vi "workbook add signed vba project.vi"(8 "error in (no error)":errorcluster, 9 "signature":string, 10 "vba_project":string, 11 "workbook":u32) -> (0 "error out":errorcluster, 3 "function return":u32(ring))   [LabVIEW 8.6]
doc: "lxw_error workbook_add_signed_vba_project(lxw_workbook workbook, const char *vba_project, const char *signature);"
uses:
  pending_lvxlsxwriter/xlsxwriter.dll
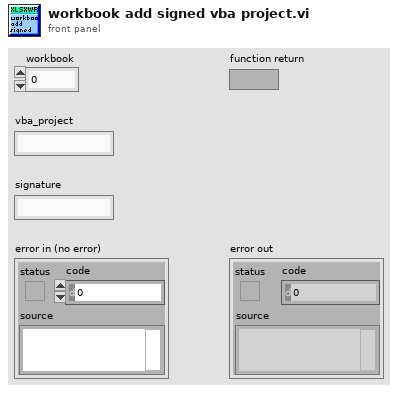
[diagram p1: front panel]
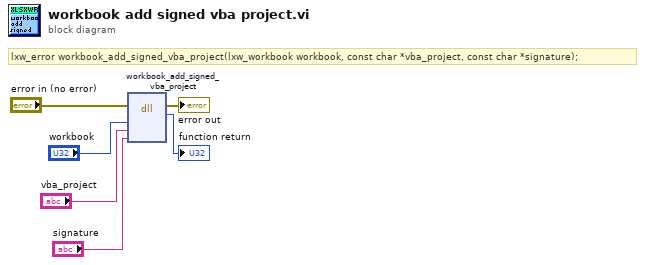
[diagram p0: block diagram]
diagram:
  # "lxw_error workbook_add_signed_vba_project(lxw_workbook workbook, const char *vba_project, const char *signature);"
  n1 = dll-call lib="C:/Users/WDAGUtilityAccount/Desktop/pending_lvxlsxwriter/xlsxwriter.*" fn="workbook_add_signed_vba_project"(error in="error in (no error)", "workbook"="workbook", "vba_project"="vba_project", "signature"="signature") -> (error out=→"error out":errorcluster, →"function return":u32)  [unwired: 5 in, 1 out]
